vi "1021th frame-Clear busy cursor.vi"(8 "error in (no error)":errorcluster, 10 "Busy cursor was set":bool) -> (0 "error out":errorcluster)   [LabVIEW 2020]
uses:
  Globals/gl_Time series viewer globals.vi
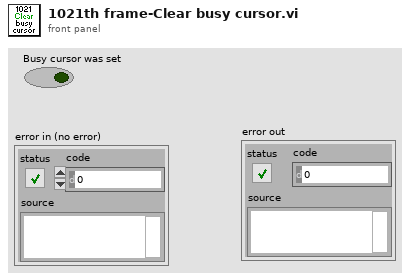
[diagram p1: front panel]
types:
  T1 = typedef "Time series viewer refs.ctl" = cluster{"This VI":refnum<vi>, "Image control":refnum<vi>, "AVI Mode ind":refnum<vi>, "Play":refnum<vi>, "Stop":refnum<vi>, "Back":refnum<vi>, "Scrollbar":refnum<vi>, "Video length info":refnum<vi>, "Expected speed values":refnum<vi>, "Intensity":refnum<vi>, "Path":refnum<vi>, "Selection sliders":refnum<vi>, "Speed Graph ref":refnum<vi>, "Frame rate set (fps)":refnum<vi>, "Number of rows to generate":refnum<vi>, "VL Image Array":refnum<vi>, "Image Scrollbar":refnum<vi>, "Channel to load":refnum<vi>, "Colour":refnum<vi>}
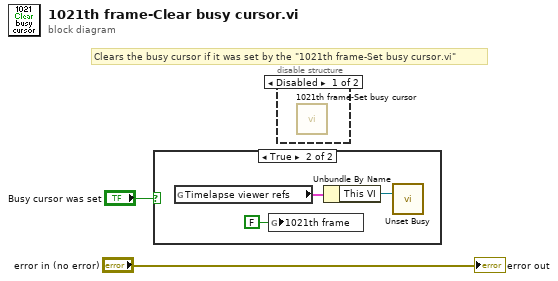
[diagram p0: block diagram]
diagram:
  # "Clears the busy cursor if it was set by the \"1021th frame-Set busy cursor.vi\""
  n1 = case shown="True" "Busy cursor was set" {
    frame False {
    }
    frame True {
      n2 = global read "gl_Time series viewer globals.vi" "Timelapse viewer refs"() -> (w5:T1)
      n3 = global write "gl_Time series viewer globals.vi" "1021th frame"(FALSE ("1021th frame")) -> ()
      n4 = Unbundle By Name(w5) -> ("This VI"=w4:refnum<vi>)
      n5 = call <vilib>:"Unset Busy.vi"("VI reference (current VI)"=w4) -> ()  [unwired: 10 in, 1 out]
    }
  }
  n6 = disable-structure shown="Disabled" {
    frame Disabled {
      n7 = call "1021th frame-Set busy cursor.vi"() -> ()  [unwired: 10 in, 2 out]
    }
    frame Enabled {
    }
  }
  "error out" <- "error in (no error)"
